vi "Write VISA & TCP_IP.vi"(8 "error in (no error)":errorcluster, 10 "VISA & TCP/IP Control":T1={"Resource Name"="COM1", "Init VISA"=TRUE, "Close VISA"=FALSE, "VISA or TCP/IP"=FALSE, "IP Address/Hostname"="10.21.163.30"}, 11 "PicomotorAxis in":refnum<class "PicomotorController.lvclass">) -> (0 "error out":errorcluster, 3 "PicomotorAxis out":refnum<class "PicomotorController.lvclass">)   [LabVIEW 2020, in "PicomotorController.lvclass"]
uses:
  PicomotorController.lvclass
  VISA & TCPIP Control.ctl
  PicomotorController.lvclass/PicomotorController.ctl
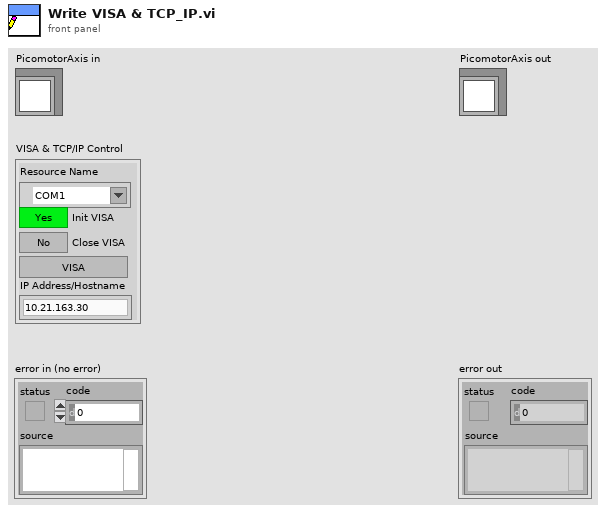
[diagram p1: front panel]
types:
  T1 = typedef "VISA & TCPIP Control.ctl" = cluster{"Resource Name":refnum<visa-resource-name>, "Init VISA":bool, "Close VISA":bool, "VISA or TCP/IP":bool, "IP Address/Hostname":string}
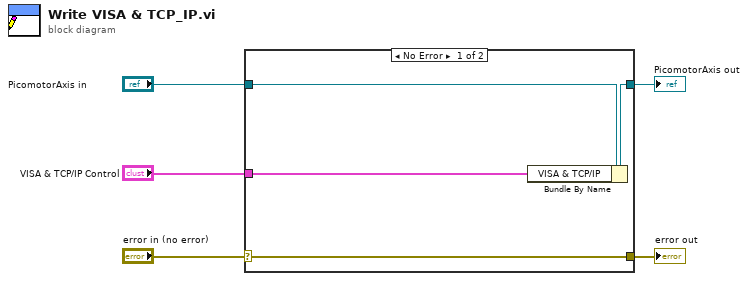
[diagram p0: block diagram]
diagram:
  n1 = case shown="No Error" "error in (no error)" {
    selector: "error in (no error)" -> [w9 w10]
    tunnel: [w9 w10] -> w4
    tunnel: [w7 w11] -> w2
    tunnel: "PicomotorAxis in" -> [w8 w11]
    tunnel: "VISA & TCP/IP Control" -> [w6 _]
    frame No Error {
      n2 = Bundle By Name(cluster=w8, "VISA & TCP/IP"=w6) -> (w7:refnum<class "PicomotorController.lvclass">)
    }
    frame Error {
    }
  }
  "error out" <- w4
  "PicomotorAxis out" <- w2
